vi "niDTS WLAN UTIL HT-MCS to NSS.vi"(10 "HT MCS":i32) -> (2 "NSS":i32)   [LabVIEW 2015, in "niDTS WLAN.lvlib"]
uses:
  niDTS WLAN.lvlib
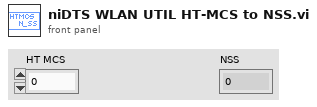
[diagram p1: front panel]
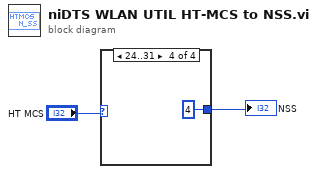
[diagram p0: block diagram]
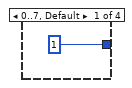
[diagram p2: hidden frame]
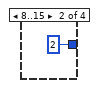
[diagram p3: hidden frame]
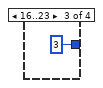
[diagram p4: hidden frame]
diagram:
  n1 = case shown="24..31" "HT MCS" {
    tunnel: [1 ("NSS") 2 ("NSS") 3 ("NSS") 4 ("NSS")] -> w1
    frame 0..7, Default {
    }
    frame 8..15 {
    }
    frame 16..23 {
    }
    frame 24..31 {
    }
  }
  "NSS" <- w1
